vi "GUI Write Sampling Status.vi"(7 "status label":string="stat3", 8 "error in":errorcluster, 10 "total samples":i64, 11 "data":T1) -> (0 "error out":errorcluster)   [LabVIEW 2018]
doc: "Updates status of sampling. Can generate error, but will exdcute even with input error."
uses:
  adc/ADC Data Packet.ctl
  varilib/SGUI Assign Multiple Strings With Tags By Label.vi
  varilib/varilib.lvlib
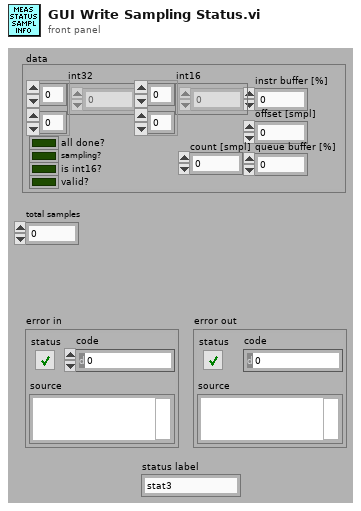
[diagram p1: front panel]
types:
  T1 = typedef "ADC Data Packet.ctl" = cluster{"int32":i32[][], "int16":i16[][], "offset [smpl]":i64, "count [smpl]":i32, "is int16?":bool, "all done?":bool, "sampling?":bool, "instr buffer [%]":dbl, "queue buffer [%]":dbl, "valid?":bool}
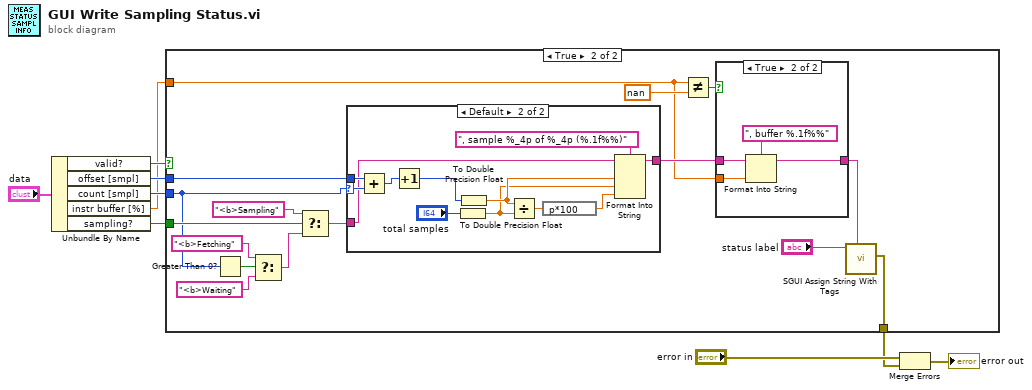
[diagram p0: block diagram]
diagram:
  n1 = Unbundle By Name("data") -> ("valid?"=w5:bool, "offset [smpl]"=w2:i64, "count [smpl]"=w3:i32, "instr buffer [%]"=w1:dbl, "sampling?"=w4:bool)
  n2 = case shown="True" w5 {
    tunnel: [_ w22] -> w7
    tunnel: w4 -> [_ w21]
    tunnel: w3 -> [_ w14]
    tunnel: w2 -> [_ w15]
    tunnel: w1 -> [_ w10]
    frame False {
    }
    frame True {
      n3 = Greater Than 0?(x=w14) -> (x > 0?=w18:bool)
      n4 = Select(t="<b>Fetching" ("format string"), s=w18, f="<b>Waiting" ("format string")) -> (s? t:f=w19:string)
      n5 = Select(t="<b>Sampling" ("format string"), s=w21, f=w19) -> (s? t:f=w11:string)
      n6 = case shown="Default" w14 {
        selector: w14 -> [_ w40]
        tunnel: [w31 w42] -> w25
        tunnel: w15 -> [_ w41]
        tunnel: w11 -> [w31 w34]
        frame 0 {
        }
        frame Default {
          n7 = Add(x=w41, y=w40) -> (x+y=w39:i64)
          n8 = Increment(x=w39) -> (x+1=w37:i64)
          n9 = To Double Precision Float(number="total samples") -> (double precision float=w32:dbl)
          n10 = To Double Precision Float(number=w37) -> (double precision float=w33:dbl)
          n11 = Divide(x=w33, y=w32) -> (x/y=w36:dbl)
          n12 = expression code="p*100"(w36) -> (w35:dbl)
          n13 = Format Into String(format string=", sample %_4p of %_4p (%.1f%%)", initial string=w34, w33, w32, w35) -> (resulting string=w42:string)  [unwired: 1 in, 1 out]
        }
      }
      n14 = Not Equal?(x=w10, y=nan) -> (x != y?=w13:bool)
      n15 = case shown="True" w13 {
        tunnel: w25 -> [w26 w29]
        tunnel: [w26 w28] -> w24
        tunnel: w10 -> [_ w27]
        frame False {
        }
        frame True {
          n16 = Format Into String(format string=", buffer %.1f%%", initial string=w29, w27) -> (resulting string=w28:string)  [unwired: 1 in, 1 out]
        }
      }
      n17 = call-poly "SGUI Assign String With Tags.vi"("label(s) (empty)"="status label", "string (empty)"=w24) -> ("error out"=w22:errorcluster)  [unwired: 8 in, 1 out]
    }
  }
  n18 = Merge Errors("error in", w7) -> (→"error out":errorcluster)
